vi "Alert Number.vi"(8 "error in (no error)":errorcluster, 10 "Numeric":dbl, 11 "Callback Consumer in":refnum<class "Callback Consumer.lvclass">) -> (0 "error out":errorcluster, 3 "Callback Consumer out":refnum<class "Callback Consumer.lvclass">)   [LabVIEW 2020, in "Callback Consumer.lvclass"]
uses:
  Callback Consumer.lvclass
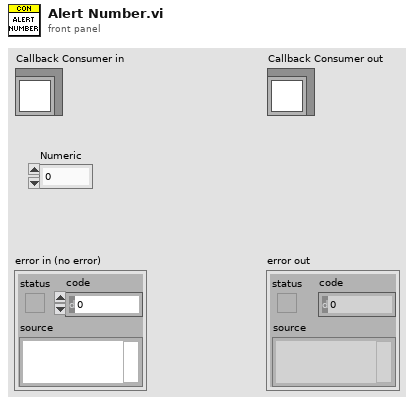
[diagram p1: front panel]
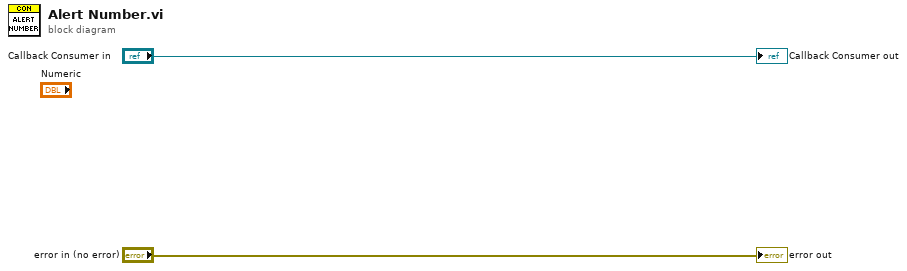
[diagram p0: block diagram]
diagram:
  "error out" <- "error in (no error)"
  "Callback Consumer out" <- "Callback Consumer in"
